vi "Contour2Poly.vi"(10 "Z":dbl, 11 "Polys":T2[](array[typedef])) -> (3 "Poly3d":cluster{T1[]}[](array[cluster]))   [LabVIEW 2014]
uses:
  TypeDefs/Poly2DwSlope.ctl
  TypeDefs/Point2DwSlope.ctl
  TypeDefs/Point3D.ctl
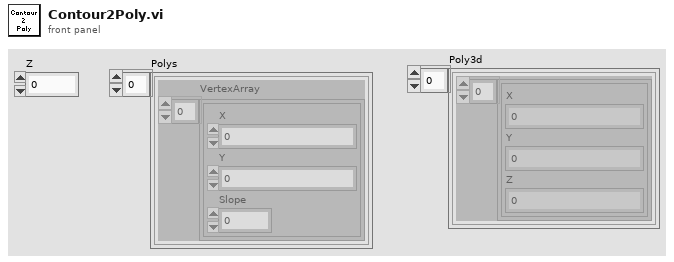
[diagram p1: front panel]
types:
  T1 = typedef "Point3D.ctl" = cluster{"X":sgl, "Y":sgl, "Z":sgl}
  T2 = typedef "Poly2DwSlope.ctl" = cluster{"VertexArray":T3[]}
  T3 = typedef "Point2DwSlope.ctl" = cluster{"X":sgl, "Y":sgl, "Slope":dbl}
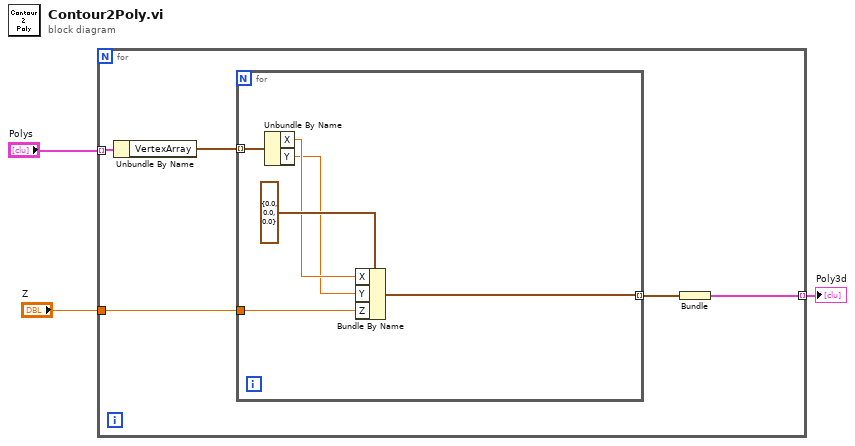
[diagram p0: block diagram]
diagram:
  n1 = for {
    tunnel: "Polys" -> [w8] mode=indexing
    tunnel: "Z" -> [w6]
    tunnel: [w4] -> w1 mode=indexing
    n2 = Unbundle By Name(w8) -> ("VertexArray"=w7:T3[])
    n3 = for {
      tunnel: w7 -> [w14] mode=indexing
      tunnel: w6 -> [w10]
      tunnel: [w9] -> w5 mode=indexing
      n4 = Unbundle By Name(w14) -> ("X"=w12:sgl, "Y"=w11:sgl)
      n5 = Bundle By Name(cluster=T1 {"X"=0.0, "Y"=0.0, "Z"=0.0} ("Point3D"), "X"=w12, "Y"=w11, "Z"=w10) -> (w9:T1)
    }
    n6 = Bundle(w5) -> (w4:cluster{T1[]})  [unwired: 1 in]
  }
  "Poly3d" <- w1
